vi "Untitled 5.vi"() -> ()   [LabVIEW 2018]
uses:
  <vilib>/express/express arith-compare/Formula/XNode/ExpressFormulaBlockNode.xnode
panel:
  out "x + iy 2":cdb
  out "x + iy":cdb
  in  "c":dbl
  in  "b":dbl
  in  "a":dbl
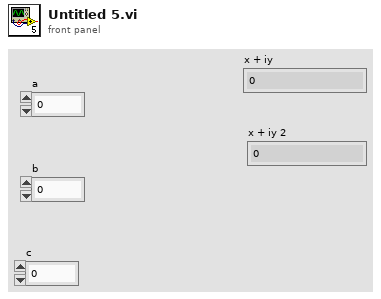
[diagram p1: front panel]
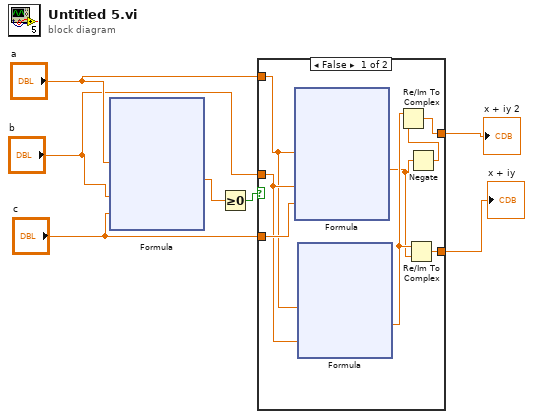
[diagram p0: block diagram]
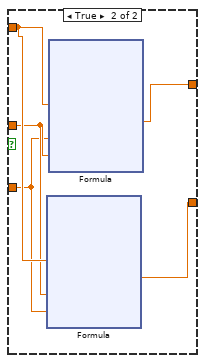
[diagram p2: hidden frame]
diagram:
  n1 = xnode "Formula"("X1"="a", "X2"="b", "X3"="c") -> ("Result"=w6:dbl)  [unwired: 1 in, 1 out]
  n2 = Greater Or Equal To 0?(x=w6) -> (x >= 0?=w7:bool)
  n3 = case shown="False" w7 {
    tunnel: "a" -> [w12 w41]
    tunnel: "b" -> [w14 w40]
    tunnel: "c" -> [w15 w39]
    tunnel: [w11 w42] -> w1
    tunnel: [w13 w38] -> w3
    frame False {
      n4 = xnode "Formula"("X1"=w12, "X2"=w14, "X3"=w15) -> ("Result"=w9:dbl)  [unwired: 1 in, 1 out]
      n5 = xnode "Formula"("X1"=w12, "X2"=w14) -> ("Result"=w10:dbl)  [unwired: 1 in, 1 out]
      n6 = Re/Im To Complex(1:w9, 2:w10) -> (0:w13:cdb)
      n7 = Negate(x=w9) -> (-x=w8:dbl)
      n8 = Re/Im To Complex(1:w8, 2:w10) -> (0:w11:cdb)
    }
    frame True {
      n9 = xnode "Formula"("X1"=w41, "X2"=w40, "X3"=w39) -> ("Result"=w38:dbl)  [unwired: 1 in, 1 out]
      n10 = xnode "Formula"("X1"=w41, "X3"=w39, "X2"=w40) -> ("Result"=w42:dbl)  [unwired: 1 in, 1 out]
    }
  }
  "x + iy" <- w3
  "x + iy 2" <- w1
